vi "PH DCT Imagehash.vi"(11 "Image Path":path) -> (3 "DCT phash":u64 format="%x")   [LabVIEW 2014, in "Perceptual Hash Comparison.lvclass"]
uses:
  Perceptual Hash Comparison.lvclass
  Perceptual Hash Comparison/phash DLL/pHash.dll
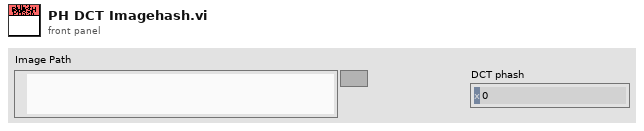
[diagram p1: front panel]
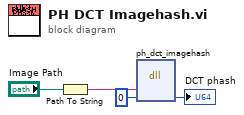
[diagram p0: block diagram]
diagram:
  n1 = Path To String(path="Image Path") -> (string=w2:string)
  n2 = dll-call lib="D:/Code/LabVIEW Reddit Coding Challenge - June 2021/Perceptual Hash Comparison/phash DLL/pHash.dll" fn="ph_dct_imagehash"("file"=w2, "hash"=u64 0) -> ("hash"=→"DCT phash":u64)  [unwired: 5 in, 2 out]
